vi "Get Config.vi"(8 "error in (no error)":errorcluster, 11 "DeployTCPResource in":refnum<class "TCPResource.lvclass">) -> (0 "error out":errorcluster, 2 "Config":T1[](array[typedef]), 3 "DeployTCPResource out":refnum<class "TCPResource.lvclass">)   [LabVIEW 2020, in "PicoG-Core.lvlib" / "TCPResource.lvclass"]
uses:
  TCPResource.lvclass
  TCPResource.lvclass/TCPResource.ctl
  Resource/Config Item.ctl
  Resource/Resource.lvclass
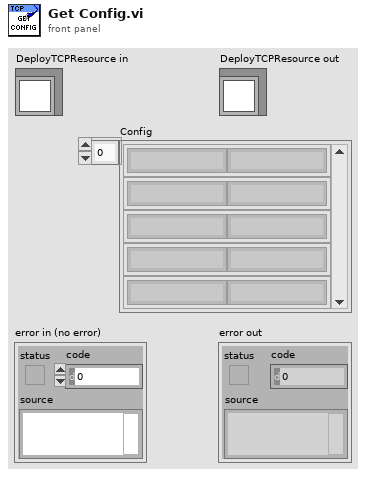
[diagram p1: front panel]
types:
  T1 = typedef "PicoG-Core.lvlib/Resource.lvclass/Config Item.ctl" = cluster{"Key":string, "Value":string}
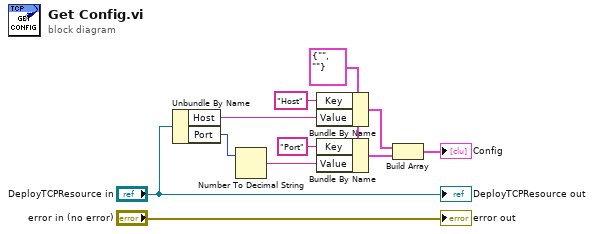
[diagram p0: block diagram]
diagram:
  w8 = T1 {"Key"="", "Value"=""} ("Config Item")
  n1 = Unbundle By Name("DeployTCPResource in") -> ("Host"=w2:string, "Port"=w9:u16)
  n2 = Number To Decimal String(number=w9) -> (decimal integer string=w3:string)  [unwired: 1 in]
  n3 = Bundle By Name(cluster=w8, "Key"="Host", "Value"=w2) -> (w5:T1)
  n4 = Bundle By Name(cluster=w8, "Key"="Port", "Value"=w3) -> (w4:T1)
  n5 = Build Array(w5, w4) -> (→"Config":T1[])
  "error out" <- "error in (no error)"
  "DeployTCPResource out" <- "DeployTCPResource in"
